vi "test_F9P_fgv-ver.vi"() -> ()   [LabVIEW 2019] (continued)
,087,42,09,44,196,27,11,77,034,40,7*7E\r\n$GAGSV,3,2,09,12,32,114,27,18,55,286,35,19,18,042,34,25,01,241,,7*7A\r\n$GAGSV,3,3,09,36,34,314,31,7*4C\r\n$GAGSV,3,1,09,02,04,288,,04,68,087,35,09,44,196,24,11,77,034,33,2*7C\r\n$GAGSV,3,2,09,12,32,114,24,18,55,286,44,19,18,042,25,25,01,241,,2*7A\r\n$GAGSV,3,3,09,36,34,314,18,2*42\r\n$GBGSV,4,1,13,04,35,133,,05,09,257,,06,27,182,,07,09,201,,1*7B\r\n$GBGSV,4,2,13,08,65,355,43,09,07,194,,10,16,222,19,11,38,142,31,1*7D\r\n$GBGSV,4,3,13,13,50,314,24,14,77,038,44,28,58,310,36,33,72,237,39,1*73\r\n$GBGSV,4,4,13,34,13,141,,1*45\r\n$GBGSV,4,1,13,04,35,133,,05,09,257,,06,27,182,,07,09,201,,3*79\r\n$GBGSV,4,2,13,08,65,355,33,09,07,194,,10,16,222,20,11,38,142,26,3*74\r\n$GBGSV,4,3,13,13,50,314,21,14,77,038,40,28,58,310,,33,72,237,,3*7F\r\n$GBGSV,4,4,13,34,13,141,,3*47\r\n$GNGLL,3723.60163,N,12656.93152,E,064153.00,A,A*7F\r\n$GNRMC,064154.00,A,3723.60205,N,12656.93230,E,2.863,60.24,250720,,,A,V*3C\r\n$GNVTG,60.24,T,,M,2.863,N,5.302,K,A*18\r\n$GNGGA,064154.00,3723.60205,N,12656.93230,E,1,12,0.62,58.0,M,18.5,M,,*7F\r\n$GNGSA,A,3,17,19,06,05,02,12,09,,,,,,1.11,0.62,0.92,1*0A\r\n$GNGSA,A,3,85,70,71,72,,,,,,,,,1.11,0.62,0.92,2*05\r\n$GNGSA,A,3,36,19,11,04,09,12,,,,,,,1.11,0.62,0.92,3*0E\r\n$GNGSA,A,3,28,14,13,11,33,08,10,,,,,,1.11,0.62,0.92,4*0E\r\n$GPGSV,4,1,13,02,65,334,44,04,08,037,25,05,48,261,38,06,58,076,46,1*66\r\n$GPGSV,4,2,13,07,06,105,,09,38,057,41,12,18,263,25,13,07,191,,1*66\r\n$GPGSV,4,3,13,17,20,157,31,19,38,161,27,25,11,294,,29,06,323,,1*63\r\n$GPGSV,4,4,13,30,01,134,,1*52\r\n$GPGSV,4,1,13,02,65,334,,04,08,037,18,05,48,261,36,06,58,076,31,6*61\r\n$GPGSV,4,2,13,07,06,105,,09,38,057,40,12,18,263,18,13,07,191,,6*6E\r\n$GPGSV,4,3,13,17,20,157,18,19,38,161,,25,11,294,,29,06,323,,6*6A\r\n$GPGSV,4,4,13,30,01,134,,6*55\r\n$GLGSV,2,1,06,70,55,030,30,71,68,223,39,72,17,216,32,84,09,133,11,1*78\r\n$GLGSV,2,2,06,85,63,111,36,86,51,337,,1*7F\r\n$GLGSV,2,1,06,70,55,030,,71,68,223,31,72,17,216,19,84,09,133,10,3*79\r\n$GLGSV,2,2,06,85,63,111,26,86,51,337,,3*7C\r\n$GAGSV,3,1,09,02,04,288,09,04,68,087,41,09,44,196,27,11,77,034,37,7*74\r\n$GAGSV,3,2,09,12,32,114,26,18,55,286,37,19,17,042,31,25,01,241,,7*73\r\n$GAGSV,3,3,09,36,34,314,25,7*49\r\n$GAGSV,3,1,09,02,04,288,,04,68,087,38,09,44,196,24,11,77,034,32,2*70\r\n$GAGSV,3,2,09,12,32,114,26,18,55,286,42,19,17,042,32,25,01,241,,2*77\r\n$GAGSV,3,3,09,36,34,314,18,2*42\r\n$GBGSV,4,1,13,04,35,133,,05,09,257,,06,27,182,,07,09,201,,1*7B\r\n$GBGSV,4,2,13,08,65,355,41,09,07,194,,10,16,222,19,11,38,142,35,1*7B\r\n$GBGSV,4,3,13,13,50,314,25,14,77,038,42,28,58,310,38,33,72,237,38,1*7B\r\n$GBGSV,4,4,13,34,13,141,,1*45\r\n$GBGSV,4,1,13,04,35,133,,05,09,257,,06,27,182,,07,09,201,,3*79\r\n$GBGSV,4,2,13,08,65,355,33,09,07,194,,10,16,222,20,11,38,142,35,3*76\r\n$GBGSV,4,3,13,13,50,314,21,14,77,038,38,28,58,310,,33,72,237,,3*70\r\n$GBGSV,4,4,13,34,13,141,,3*47\r\n$GNGLL,3723.60205,N,12656.93230,E,064154.00,A,A*7C\r\n$GNRMC,064155.00,A,3723.60234,N,12656.93308,E,2.533,62.68,250720,,,A,V*37\r\n$GNVTG,62.68,T,,M,2.533,N,4.692,K,A*17\r\n$GNGGA,064155.00,3723.60234,N,12656.93308,E,1,12,0.73,57.4,M,18.5,M,,*7D\r\n$GNGSA,A,3,17,19,06,05,02,12,09,,,,,,1.21,0.73,0.97,1*0C\r\n$GNGSA,A,3,85,70,71,72,,,,,,,,,1.21,0.73,0.97,2*03\r\n$GNGSA,A,3,36,19,11,04,09,12,,,,,,,1.21,0.73,0.97,3*08\r\n$GNGSA,A,3,28,14,13,11,33,08,10,,,,,,1.21,0.73,0.97,4*08\r\n$GPGSV,4,1,13,02,65,334,44,04,08,037,24,05,48,261,41,06,58,076,44,1*6B\r\n$GPGSV,4,2,13,07,06,105,,09,38,057,45,12,18,263,25,13,08,191,,1*6D\r\n$GPGSV,4,3,13,17,20,157,31,19,38,161,27,25,11,294,,29,06,323,,1*63\r\n$GPGSV,4,4,13,30,01,134,,1*52\r\n$GPGSV,4,1,13,02,65,334,,04,08,037,19,05,48,261,36,06,58,076,32,6*63\r\n$GPGSV,4,2,13,07,06,105,,09,38,057,38,12,18,263,19,13,08,191,,6*6F\r\n$GPGSV,4,3,13,17,20,157,17,19,38,161,,25,11,294,,29,06,323,,6*65\r\n$GPGSV,4,4,13,30,01,134,,6*55\r\n$GLGSV,2,1,06,70,55,030,29,71,68,223,37,72,17,216,31,84,09,133,10,1*7C\r\n$GLGSV,2,2,06,85,63,111,32,86,51,337,,1*7B\r\n$GLGSV,2,1,06,70,55,030,,71,68,223,30,72,17,216,19,84,09,133,08,3*71\r\n$GLGSV,2,2,06,85,63,111,26,86,51,337,,3*7C\r\n$GAGSV,3,1,09,02,04,288,10,04,68,087,39,09,44,196,27,11,77,034,38,7*7C\r\n$GAGSV,3,2,09,12,32,114,25,18,55,286,39,19,17,042,27,25,01,241,,7*79\r\n$GAGSV,3,3,09,36,34,314,26,7*4A\r\n$GAGSV,3,1,09,02,04,288,,04,68,087,33,09,44,196,25,11,77,034,35,2*7D\r\n$GAGSV,3,2,09,12,32,114,25,18,55,286,42,19,17,042,30,25,01,241,,2*76\r\n$GAGSV,3,3,09,36,34,314,19,2*43\r\n$GBGSV,4,1,13,04,35,133,,05,09,257,,06,27,182,,07,09,201,,1*7B\r\n$GBGSV,4,2,13,08,65,355,42,09,07,194,,10,16,222,19,11,38,142,23,1*7F\r\n$GBGSV,4,3,13,13,50,314,25,14,77,038,41,28,58,310,32,33,72,237,40,1*7D\r\n$GBGSV,4,4,13,34,13,141,,1*45\r\n$GBGSV,4,1,13,04,35,133,,05,09,257,,06,27,182,,07,09,201,,3*79\r\n$GBGSV,4,2,13,08,65,355,34,09,07,194,,10,16,222,21,11,38,142,28,3*7C\r\n$GBGSV,4,3,13,13,50,314,21,14,77,038,41,28,58,310,,33,72,237,,3*7E\r\n$GBGSV,4,4,13,34,13,141,,3*47\r\n$GNGLL,3723.60234,N,12656.93308,E,064155.00,A,A*75\r\n$GNRMC,064156.00,A,3723.60265,N,12656.93385,E,2.612,63.63,250720,,,A,V*3F\r\n$GNVTG,63.63,T,,M,2.612,N,4.837,K,A*1C\r\n$GNGGA,064156.00,3723.60265,N,12656.93385,E,1,12,0.67,56.6,M,18.5,M,,*79\r\n$GNGSA,A,3,17,19,06,05,02,12,09,,,,,,1.14,0.67,0.93,1*0B\r\n$GNGSA,A,3,85,70,71,72,,,,,,,,,1.14,0.67,0.93,2*04\r\n$GNGSA,A,3,36,19,11,04,09,12,,,,,,,1.14,0.67,0.93,3*0F\r\n$GNGSA,A,3,28,14,13,11,33,08,10,,,,,,1.14,0.67,0.93,4*0F\r\n$GPGSV,4,1,13,02,65,334,46,04,08,037,23,05,48,261,39,06,58,076,42,1*67\r\n$GPGSV,4,2,13,07,06,105,,09,38,057,46,12,18,263,25,13,08,191,,1*6E\r\n$GPGSV,4,3,13,17,20,157,37,19,38,161,37,25,11,294,,29,06,323,,1*64\r\n$GPGSV,4,4,13,30,01,134,,1*52\r\n$GPGSV,4,1,13,02,65,334,,04,08,037,19,05,48,261,37,06,58,076,31,6*61\r\n$GPGSV,4,2,13,07,06,105,,09,38,057,39,12,18,263,19,13,08,191,,6*6E\r\n$GPGSV,4,3,13,17,20,157,21,19,38,161,,25,11,294,,29,06,323,,6*60\r\n$GPGSV,4,4,13,30,01,134,,6*55\r\n$GLGSV,2,1,06,70,55,030,36,71,68,223,42,72,17,216,25,84,09,133,10,1*75\r\n$GLGSV,2,2,06,85,63,111,32,86,51,337,,1*7B\r\n$GLGSV,2,1,06,70,55,030,,71,68,223,28,72,17,216,20,84,09,133,11,3*7A\r\n$GLGSV,2,2,06,85,63,111,35,86,51,337,,3*7E\r\n$GAGSV,3,1,09,02,04,288,08,04,68,087,40,09,44,196,26,11,77,034,38,7*7A\r\n$GAGSV,3,2,09,12,32,114,31,18,55,286,41,19,17,042,32,25,01,241,,7*77\r\n$GAGSV,3,3,09,36,34,314,28,7*44\r\n$GAGSV,3,1,09,02,04,288,,04,68,087,36,09,44,196,25,11,77,034,34,2*79\r\n$GAGSV,3,2,09,12,32,114,25,18,55,286,44,19,17,042,32,25,01,241,,2*72\r\n$GAGSV,3,3,09,36,34,314,,2*4B\r\n$GBGSV,4,1,13,04,35,133,,05,09,257,,06,27,182,,07,09,201,,1*7B\r\n$GBGSV,4,2,13,08,65,355,44,09,07,194,,10,16,222,19,11,38,142,30,1*7B\r\n$GBGSV,4,3,13,13,50,314,31,14,77,038,43,28,58,310,43,33,72,237,41,1*7D\r\n$GBGSV,4,4,13,34,13,141,,1*45\r\n$GBGSV,4,1,13,04,35,133,,05,09,257,,06,27,182,,07,09,201,,3*79\r\n$GBGSV,4,2,13,08,65,355,35,09,07,194,,10,16,222,22,11,38,142,33,3*74\r\n$GBGSV,4,3,13,13,50,314,,14,77,038,39,28,58,310,,33,72,237,,3*72\r\n$GBGSV,4,4,13,34,13,141,,3*47\r\n$GNGLL,3723.60265,N,12656.93385,E,064156.00,A,A*77\r\n$GNRMC,064157.00,A,3723.60305,N,12656.93457,E,2.616,59.21,250720,,,A,V*3A\r\n$GNVTG,59.21,T,,M,2.616,N,4.845,K,A*12\r\n$GNGGA,064157.00,3723.60305,N,12656.93457,E,1,12,0.64,56.0,M,18.5,M,,*72\r\n$GNGSA,A,3,17,19,06,05,02,12,09,,,,,,1.12,0.64,0.92,1*0F\r\n$GNGSA,A,3,85,70,71,72,,,,,,,,,1.12,0.64,0.92,2*00\r\n$GNGSA,A,3,36,19,11,04,09,12,,,,,,,1.12,0.64,0.92,3*0B\r\n$GNGSA,A,3,28,14,13,11,33,08,10,,,,,,1.12,0.64,0.92,4*0B\r\n$GPGSV,4,1,13,02,65,334,47,04,08,037,22,05,48,261,35,06,58,076,43,1*6A\r\n$GPGSV,4,2,13,07,06,105,,09,38,057,45,12,18,263,,13,08,191,,1*6A\r\n$GPGSV,4,3,13,17,20,157,34,19,38,161,36,25,11,294,17,29,06,323,,1*60\r\n$GPGSV,4,4,13,30,01,134,,1*52\r\n$GPGSV,4,1,13,02,65,334,,04,08,037,20,05,48,261,39,06,58,076,34,6*60\r\n$GPGSV,4,2,13,07,06,105,,09,38,057,41,12,18,263,18,13,08,191,,6*60\r\n$GPGSV,4,3,13,17,20,157,30,19,38,161,,25,11,294,,29,06,323,,6*60\r\n$GPGSV,4,4,13,30,01,134,,6*55\r\n$GLGSV,2,1,06,70,55,030,29,71,68,223,42,72,17,216,25,84,09,133,09,1*73\r\n$GLGSV,2,2,06,85,63,111,30,86,51,337,,1*79\r\n$GLGSV,2,1,06,70,55,030,,71,68,223,28,72,17,216,21,84,09,133,11,3*7B\r\n$GLGSV,2,2,06,85,63,111,27,86,51,337,,3*7D\r\n$GAGSV,3,1,09,02,04,288,07,04,68,087,40,09,44,196,31,11,77,034,39,7*72\r\n$GAGSV,3,2,09,12,32,114,31,18,55,286,40,19,17,042,28,25,01,241,,7*7D\r\n$GAGSV,3,3,09,36,34,314,35,7*48\r\n$GAGSV,3,1,09,02,04,288,,04,68,087,33,09,44,196,30,11,77,034,36,2*7A\r\n$GAGSV,3,2,09,12,32,114,24,18,55,286,46,19,17,042,32,25,01,241,,2*71\r\n$GAGSV,3,3,09,36,34,314,,2*4B\r\n$GBGSV,4,1,13,04,35,133,,05,09,257,,06,27,182,,07,09,201,,1*7B\r\n$GBGSV,4,2,13,08,65,355,41,09,07,194,,10,16,222,20,11,38,142,28,1*7D\r\n$GBGSV,4,3,13,13,50,314,31,14,77,038,41,28,58,310,40,33,72,237,42,1*7F\r\n$GBGSV,4,4,13,34,13,141,,1*45\r\n$GBGSV,4,1,13,04,35,133,,05,09,257,,06,27,182,,07,09,201,,3*79\r\n$GBGSV,4,2,13,08,65,355,37,09,07,194,,10,16,222,22,11,38,142,,3*76\r\n$GBGSV,4,3,13,13,50,314,28,14,77,038,41,28,58,310,,33,72,237,,3*77\r\n$GBGSV,4,4,13,34,13,141,,3*47\r\n$GNGLL,3723.60305,N,12656.93457,E,064157.00,A,A*79\r\n$GNRMC,064158.00,A,3723.60345,N,12656.93529,E,2.695,59.49,250720,,,A,V*3C\r\n$GNVTG,59.49,T,,M,2.695,N,4.991,K,A*1F\r\n$GNGGA,064158.00,3723.60345,N,12656.93529,E,1,12,0.67,55.4,M,18.5,M,,*75\r\n$GNGSA,A,3,17,19,06,05,02,12,09,,,,,,1.12,0.67,0.90,1*0E\r\n$GNGSA,A,3,85,70,71,72,,,,,,,,,1.12,0.67,0.90,2*01\r\n$GNGSA,A,3,36,19,11,04,09,12,,,,,,,1.12,0.67,0.90,3*0A\r\n$GNGSA,A,3,28,14,13,11,33,08,10,,,,,,1.12,0.67,0.90,4*0A\r\n$GPGSV,4,1,13,02,65,334,47,04,08,037,22,05,48,261,37,06,58,076,38,1*64\r\n$GPGSV,4,2,13,07,06,105,,09,38,057,45,12,18,263,31,13,08,191,,1*68\r\n$GPGSV,4,3,13,17,19,158,29,19,38,161,27,25,11,294,20,29,06,323,,1*6D\r\n$GPGSV,4,4,13,30,01,134,,1*52\r\n$GPGSV,4,1,13,02,65,334,,04,08,037,19,05,48,261,38,06,58,076,24,6*6A\r\n$GPGSV,4,2,13,07,06,105,,09,38,057,41,12,18,263,20,13,08,191,,6*6B\r\n$GPGSV,4,3,13,17,19,158,22,19,38,161,,25,11,294,,29,06,323,,6*66\r\n$GPGSV,4,4,13,30,01,134,,6*55\r\n$GLGSV,2,1,06,70,55,030,33,71,68,223,39,72,17,216,30,84,09,133,11,1*79\r\n$GLGSV,2,2,06,85,63,111,32,86,51,337,,1*7B\r\n$GLGSV,2,1,06,70,55,030,,71,68,223,28,72,17,216,20,84,09,133,12,3*79\r\n$GLGSV,2,2,06,85,63,111,26,86,51,337,,3*7C\r\n$GAGSV,3,1,09,02,04,288,08,04,68,087,38,09,44,196,29,11,77,034,38,7*7A\r\n$GAGSV,3,2,09,12,32,114,29,18,55,286,42,19,17,042,26,25,01,241,,7*78\r\n$GAGSV,3,3,09,36,34,314,41,7*4B\r\n$GAGSV,3,1,09,02,04,288,,04,68,087,31,09,44,196,20,11,77,034,36,2*79\r\n$GAGSV,3,2,09,12,32,114,31,18,55,286,44,19,17,042,25,25,01,241,,2*71\r\n$GAGSV,3,3,09,36,34,314,37,2*4F\r\n$GBGSV,4,1,13,04,35,133,,05,09,257,,06,27,182,,07,09,201,,1*7B\r\n$GBGSV,4,2,13,08,65,355,42,09,07,194,,10,16,222,21,11,38,142,27,1*70\r\n$GBGSV,4,3,13,13,50,314,39,14,77,038,40,28,58,310,34,33,72,237,41,1*76\r\n$GBGSV,4,4,13,34,13,141,,1*45\r\n$GBGSV,4,1,13,04,35,133,,05,09,257,,06,27,182,,07,09,201,,3*79\r\n$GBGSV,4,2,13,08,65,355,35,09,07,194,,10,16,222,22,11,38,142,26,3*70\r\n$GBGSV,4,3,13,13,50,314,34,14,77,038,38,28,58,310,,33,72,237,,3*74\r\n$GBGSV,4,4,13,34,13,141,,3*47\r\n$GNGLL,3723.60345,N,12656.93529,E,064158.00,A,A*7A\r\n$GNRMC,064159.00,A,3723.60384,N,12656.93601,E,2.607,56.76,250720,,,A,V*31\r\n$GNVTG,56.76,T,,M,2.607,N,4.827,K,A*1B\r\n$GNGGA,064159.00,3723.60384,N,12656.93601,E,1,12,0.67,54.9,M,18.5,M,,*7C\r\n$GNGSA,A,3,17,19,06,05,02,12,09,,,,,,1.14,0.67,0.93,1*0B\r\n$GNGSA,A,3,85,70,71,72,,,,,,,,,1.14,0.67,0.93,2*04\r\n$GNGSA,A,3,36,19,11,04,09,12,,,,,,,1.14,0.67,0.93,3*0F\r\n$GNGSA,A,3,28,14,13,11,33,08,10,,,,,,1.14,0.67,0.93,4*0F\r\n$GPGSV,4,1,13,02,65,334,49,04,08,037,22,05,48,261,41,06,58,076,39,1*6A\r\n$GPGSV,4,2,13,07,06,105,,09,38,057,41,12,18,263,30,13,08,191,,1*6D\r\n$GPGSV,4,3,13,17,19,158,35,19,38,161,35,25,11,294,20,29,06,323,,1*63\r\n$GPGSV,4,4,13,30,01,134,,1*52\r\n$GPGSV,4,1,13,02,65,334,,04,08,037,21,05,48,261,38,06,58,076,33,6*67\r\n$GPGSV,4,2,13,07,06,105,,09,38,057,39,12,18,263,21,13,08,191,,6*65\r\n$GPGSV,4,3,13,17,19,158,29,19,38,161,,25,11,294,,29,06,323,,6*6D\r\n$GPGSV,4,4,13,30,01,134,,6*55\r\n$GLGSV,2,1,06,70,55,030,33,71,68,223,40,72,17,216,37,84,09,133,08,1*78\r\n$GLGSV,2,2,06,85,63,111,29,86,51,337,,1*71\r\n$GLGSV,2,1,06,70,55,030,,71,68,223,28,72,17,216,21,84,09,133,10,3*7A\r\n$GLGSV,2,2,06,85,63,111,25,86,51,337,,3*7F\r\n$GAGSV,3,1,09,02,04,288,09,04,68,087,38,09,44,196,29,11,77,034,38,7*7B\r\n$GAGSV,3,2,09,12,32,114,28,18,55,286,39,19,17,042,24,25,01,241,,7*77\r\n$GAGSV,3,3,09,36,34,314,34,7*49\r\n$GAGSV,3,1,09,02,04,288,,04,68,087,29,09,44,196,22,11,77,034,35,2*71\r\n$GAGSV,3,2,09,12,32,114,35,18,55,286,42,19,17,042,25,25,01,241,,2*73\r\n$GAGSV,3,3,09,36,34,314,30,2*48\r\n$GBGSV,4,1,13,04,35,133,,05,09,257,,06,27,182,,07,09,201,,1*7B\r\n$GBGSV,4,2,13,08,65,355,39,09,07,194,,10,16,222,21,11,38,142,27,1*7C\r\n$GBGSV,4,3,13,13,50,314,30,14,77,038,41,28,58,310,39,33,72,237,40,1*72\r\n$GBGSV,4,4,13,34,13,141,,1*45\r\n$GBGSV,4,1,13,04,35,133,,05,09,257,,06,27,182,,07,09,201,,3*79\r\n$GBGSV,4,2,13,08,65,355,35,09,07,194,,10,16,222,21,11,38,142,27,3*72\r\n$GBGSV,4,3,13,13,50,314,30,14,77,038,38,28,58,310,,33,72,237,,3*70\r\n$GBGSV,4,4,13,34,13,141,,3*47\r\n$GNGLL,3723.60384,N,12656.93601,E,064159.00,A,A*7F\r\n$GNRMC,064200.00,A,3723.60415,N,12656.93680,E,2.644,62.21,250720,,,A,V*3A\r\n$GNVTG,62.21,T,,M,2.644,N,4.897,K,A*12\r\n$GNGGA,064200.00,3723.60415,N,12656.93680,E,1,12,0.64,54.3,M,18.5,M,,*7C\r\n$GNGSA,A,3,17,19,06,05,02,12,09,,,,,,1.09,0.64,0.88,1*0E\r\n$GNGSA,A,3,85,70,71,72,,,,,,,,,1.09,0.64,0.88,2*01\r\n$GNGSA,A,3,36,19,11,04,09,12,,,,,,,1.09,0.64,0.88,3*0A\r\n$GNGSA,A,3,28,14,13,11,33,08,10,,,,,,1.09,0.64,0.88,4*0A\r\n$GPGSV,4,1,13,02,65,334,44,04,08,037,30,05,48,261,41,06,58,076,42,1*68\r\n$GPGSV,4,2,13,07,06,105,,09,38,057,46,12,18,263,30,13,08,191,,1*6A\r\n$GPGSV,4,3,13,17,19,158,27,19,37,161,34,25,11,294,21,29,06,323,,1*6F\r\n$GPGSV,4,4,13,30,01,134,,1*52\r\n$GPGSV,4,1,13,02,65,334,,04,08,037,20,05,48,261,35,06,58,076,29,6*60\r\n$GPGSV,4,2,13,07,06,105,,09,38,057,40,12,18,263,23,13,08,191,,6*69\r\n$GPGSV,4,3,13,17,19,158,20,19,37,161,,25,11,294,,29,06,323,,6*6B\r\n$GPGSV,4,4,13,30,01,134,,6*55\r\n$GLGSV,2,1,06,70,55,030,34,71,68,223,39,72,17,216,30,84,09,133,08,1*76\r\n$GLGSV,2,2,06,85,63,111,35,86,51,337,,1*7C\r\n$GLGSV,2,1,06,70,55,030,,71,68,223,29,72,17,216,20,84,09,133,12,3*78\r\n$GLGSV,2,2,06,85,63,111,25,86,51,337,,3*7F\r\n$GAGSV,3,1,09,02,04,288,09,04,68,087,41,09,44,196,27,11,77,034,39,7*7A\r\n$GAGSV,3,2,09,12,32,114,28,18,55,286,40,19,17,042,24,25,01,241,,7*79\r\n$GAGSV,3,3,09,36,34,314,30,7*4D\r\n$GAGSV,3,1,09,02,04,288,,04,68,087,28,09,44,196,23,11,77,034,33,2*77\r\n$GAGSV,3,2,09,12,32,114,30,18,55,286,45,19,17,042,30,25,01,241,,2*75\r\n$GAGSV,3,3,09,36,34,314,28,2*41\r\n$GBGSV,4,1,13,04,35,133,,05,09,257,,06,27,182,,07,09,201,,1*7B\r\n$GBGSV,4,2,13,08,65,355,42,09,07,194,,10,16,222,21,11,38,142,33,1*75\r\n$GBGSV,4,3,13,13,50,314,21,14,77,038,41,28,58,310,35,33,72,237,43,1*7D\r\n$GBGSV,4,4,13,34,13,141,,1*45\r\n$GBGSV,4,1,13,04,35,133,,05,09,257,,06,27,182,,07,09,201,,3*79\r\n$GBGSV,4,2,13,08,65,355,34,09,07,194,,10,16,222,19,11,38,142,32,3*7C\r\n$GBGSV,4,3,13,13,50,314,25,14,77,038,42,28,58,310,,33,72,237,,3*79\r\n$GBGSV,4,4,13,34,13,141,,3*47\r\n$GNGLL,3723.60415,N,12656.93680,E,064200.00,A,A*76\r\n$GNRMC,064201.00,A,3723.60447,N,12656.93758,E,2.481,61.92,250720,,,A,V*38\r\n$GNVTG,61.92,T,,M,2.481,N,4.594,K,A*1C\r\n$GNGGA,064201.00,3723.60447,N,12656.93758,E,1,12,0.61,53.8,M,18.5,M,,*77\r\n$GNGSA,A,3,17,19,06,05,02,12,09,,,,,,1.07,0.61,0.88,1*05\r\n$GNGSA,A,3,85,70,71,72,,,,,,,,,1.07,0.61,0.88,2*0A\r\n$GNGSA,A,3,36,19,11,04,09,12,,,,,,,1.07,0.61,0.88,3*01\r\n$GNGSA,A,3,28,14,13,11,33,08,10,,,,,,1.07,0.61,0.88,4*01\r\n$GPGSV,4,1,13,02,65,334,43,04,08,037,25,05,48,261,43,06,58,076,39,1*65\r\n$GPGSV,4,2,13,07,06,105,,09,38,057,45,12,18,263,30,13,08,191,,1*69\r\n$GPGSV,4,3,13,17,19,158,26,19,37,161,29,25,11,294,20,29,06,323,,1*63\r\n$GPGSV,4,4,13,30,01,134,,1*52\r\n$GPGSV,4,1,13,02,65,334,,04,08,037,18,05,48,261,35,06,58,076,31,6*62\r\n$GPGSV,4,2,13,07,06,105,,09,38,057,39,12,18,263,22,13,08,191,,6*66\r\n$GPGSV,4,3,13,17,19,158,19,19,37,161,,25,11,294,,29,06,323,,6*61\r\n$GPGSV,4,4,13,30,01,134,,6*55\r\n$GLGSV,2,1,06,70,55,030,34,71,68,223,41,72,17,216,30,84,09,133,10,1*70\r\n$GLGSV,2,2,06,85,63,111,33,86,51,337,,1*7A\r\n$GLGSV,2,1,06,70,55,030,,71,68,223,28,72,17,216,21,84,09,133,09,3*72\r\n$GLGSV,2,2,06,85,63,111,27,86,51,337,,3*7D\r\n$GAGSV,3,1,09,02,04,288,09,04,68,087,37,09,44,196,28,11,77,034,40,7*7A\r\n$GAGSV,3,2,09,12,32,114,28,18,55,286,37,19,17,042,24,25,01,241,,7*79\r\n$GAGSV,3,3,09,36,34,314,31,7*4C\r\n$GAGSV,3,1,09,02,04,288,,04,68,087,27,09,44,196,23,11,77,034,33,2*78\r\n$GAGSV,3,2,09,12,32,114,25,18,55,286,44,19,17,042,30,25,01,241,,2*70\r\n$GAGSV,3,3,09,36,34,314,27,2*4E\r\n$GBGSV,4,1,13,04,35,133,,05,09,257,,06,27,182,,07,09,201,,1*7B\r\n$GBGSV,4,2,13,08,65,355,42,09,07,194,,10,16,222,20,11,38,142,43,1*73\r\n$GBGSV,4,3,13,13,50,314,21,14,77,038,41,28,58,310,36,33,72,237,38,1*72\r\n$GBGSV,4,4,13,34,13,141,,1*45\r\n$GBGSV,4,1,13,04,35,133,,05,09,257,,06,27,182,,07,09,201,,3*79\r\n$GBGSV,4,2,13,08,65,355,34,09,07,194,,10,16,222,19,11,38,142,37,3*79\r\n$GBGSV,4,3,13,13,50,314,22,14,77,038,40,28,58,310,,33,72,237,,3*7C\r\n$GBGSV,4,4,13,34,13,141,,3*47\r\n$GNGLL,3723.60447,N,12656.93758,E,064201.00,A,A*74\r\n$GNRMC,064202.00,A,3723.60479,N,12656.93834,E,2.488,62.60,250720,,,A,V*34\r\n$GNVTG,62.60,T,,M,2.488,N,4.608,K,A*1D\r\n$GNGGA,064202.00,3723.60479,N,12656.93834,E,1,12,0.61,53.4,M,18.5,M,,*70\r\n$GNGSA,A,3,17,19,06,05,02,12,09,,,,,,1.07,0.61,0.88,1*05\r\n$GNGSA,A,3,85,70,71,72,,,,,,,,,1.07,0.61,0.88,2*0A\r\n$GNGSA,A,3,36,19,11,04,09,12,,,,,,,1.07,0.61,0.88,3*01\r\n$GNGSA,A,3,28,14,13,11,33,08,10,,,,,,1.07,0.61,0.88,4*01\r\n$GPGSV,4,1,13,02,65,334,43,04,08,037,25,05,48,261,40,06,58,076,38,1*67\r\n$GPGSV,4,2,13,07,06,105,,09,38,057,47,12,18,263,29,13,08,191,,1*63\r\n$GPGSV,4,3,13,17,19,158,26,19,37,161,30,25,11,294,22,29,06,323,,1*69\r\n$GPGSV,4,4,13,30,01,134,,1*52\r\n$GPGSV,4,1,13,02,65,334,,04,08,037,17,05,48,261,35,06,58,076,34,6*68\r\n$GPGSV,4,2,13,07,06,105,,09,38,057,42,12,18,263,19,13,08,191,,6*62\r\n$GPGSV,4,3,13,17,19,158,18,19,37,161,,25,11,294,,29,06,323,,6*60\r\n$GPGSV,4,4,13,30,01,134,,6*55\r\n$GLGSV,2,1,06,70,55,030,34,71,68,223,41,72,17,216,28,84,09,133,09,1*71\r\n$GLGSV,2,2,06,85,63,111,34,86,51,337,,1*7D\r\n$GLGSV,2,1,06,70,55,030,,71,68,223,28,72,17,216,21,84,09,133,11,3*7B\r\n$GLGSV,2,2,06,85,63,111,27,86,51,337,,3*7D\r\n$GAGSV,3,1,09,02,04,288,09,04,68,087,35,09,44,196,27,11,77,034,40,7*77\r\n$GAGSV,3,2,09,12,32,114,27,18,55,286,40,19,17,042,24,25,01,241,,7*76\r\n$GAGSV,3,3,09,36,34,314,25,7*49\r\n$GAGSV,3,1,09,02,04,288,,04,68,087,32,09,44,196,23,11,77,034,33,2*7C\r\n$GAGSV,3,2,09,12,32,114,25,18,55,286,46,19,17,042,,25,01,241,,2*71\r\n$GAGSV,3,3,09,36,34,314,24,2*4D\r\n$GBGSV,4,1,13,04,35,133,,05,09,257,,06,27,182,,07,09,201,,1*7B\r\n$GBGSV,4,2,13,08,65,355,41,09,07,194,,10,16,222,19,11,38,142,31,1*7F\r\n$GBGSV,4,3,13,13,50,314,21,14,77,038,42,28,58,310,33,33,72,237,41,1*7A\r\n$GBGSV,4,4,13,34,13,141,,1*45\r\n$GBGSV,4,1,13,04,35,133,,05,09,257,,06,27,182,,07,09,201,,3*79\r\n$GBGSV,4,2,13,08,65,355,32,09,07,194,,10,16,222,18,11,38,142,33,3*7A\r\n$GBGSV,4,3,13,13,50,314,21,14,77,038,36,28,58,310,,33,72,237,,3*7E\r\n$GBGSV,4,4,13,34,13,141,,3*47\r\n$GNGLL,3723.60479,N,12656.93834,E,064202.00,A,A*7F\r\n$GNRMC,064203.00,A,3723.60513,N,12656.93913,E,2.569,61.96,250720,,,A,V*38\r\n$GNVTG,61.96,T,,M,2.569,N,4.758,K,A*1D\r\n$GNGGA,064203.00,3723.60513,N,12656.93913,E,1,12,0.61,53.0,M,18.5,M,,*7C\r\n$GNGSA,A,3,17,19,06,05,02,12,09,,,,,,1.07,0.61,0.88,1*05\r\n$GNGSA,A,3,85,70,71,72,,,,,,,,,1.07,0.61,0.88,2*0A\r\n$GNGSA,A,3,36,19,11,04,09,12,,,,,,,1.07,0.61,0.88,3*01\r\n$GNGSA,A,3,28,14,13,11,33,08,10,,,,,,1.07,0.61,0.88,4*01\r\n$GPGSV,4,1,13,02,65,334,42,04,08,037,23,05,48,261,37,06,58,076,39,1*61\r\n$GPGSV,4,2,13,07,06,105,,09,38,057,46,12,18,263,28,13,08,191,,1*63\r\n$GPGSV,4,3,13,17,19,158,26,19,37,161,29,25,11,294,22,29,06,323,,1*61\r
